vi "Puzzle 24-2.vi"() -> ()   [LabVIEW 2022 SP3]
uses:
  <vilib>/gmath/zero.llb/nD Nonlinear System Solver (Formula).vi
  c09a35fd-dfb7-4751-8a6c-d1f927b46256.vi
  c23b235e-6b21-46d7-9deb-4925a2cb368b.vi
  <vilib>/gmath/NI_Gmath.lvlib
panel:
  in  "delimited string":string="65408297713475, 57213841527206, 185313960119735 @ 316, 321, 204\n185109670669244, 12706941956960, 43641783548659 @ 163, 423, 416\n57063184441840, 2848723329813, 179657077519134 @ 281, 332, 221\n93328649189759, 26248115804612, 49995133784360 @ 290, 377, 390"
  out "sum":dbl
  out "subarray":dbl[][](array[numeric])
  out "f(Zeroes)":dbl[][](array[numeric]) format="%0.2e"
  out "Zeroes 2":dbl[][](array[numeric])
  out "error":i32
  in  "index":i32
  out "Zeroes":dbl[][](array[numeric])
  out "Array":string[](array[string])
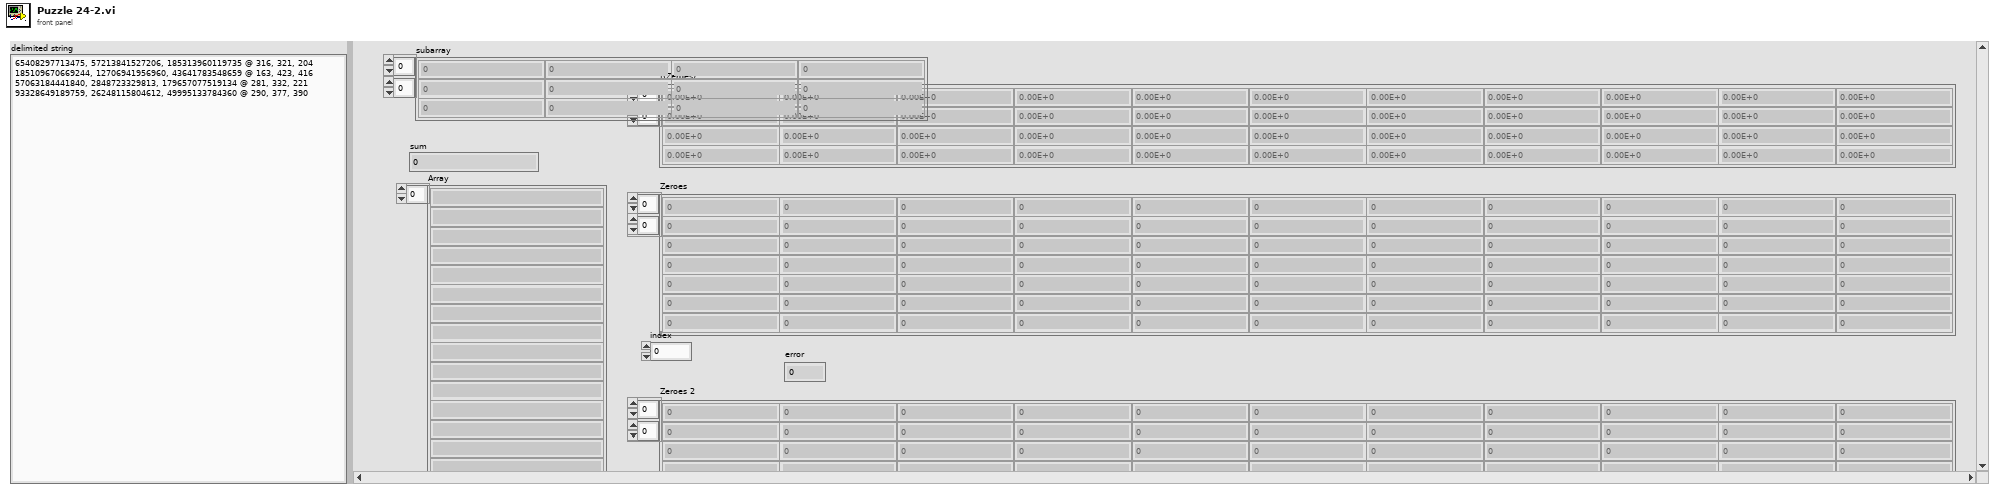
[diagram p1: front panel]
types:
  T1 = cluster{"cluster":cluster{"x":u64, "y":u64, "z":u64}, "cluster":cluster{"x":i64, "y":i64, "z":i64}}
  T2 = cluster{"cluster":cluster{"x":u64, "y":u64, "z":u64}, "cluster":cluster{"x":i64, "y":i64, "z":i64}}[]
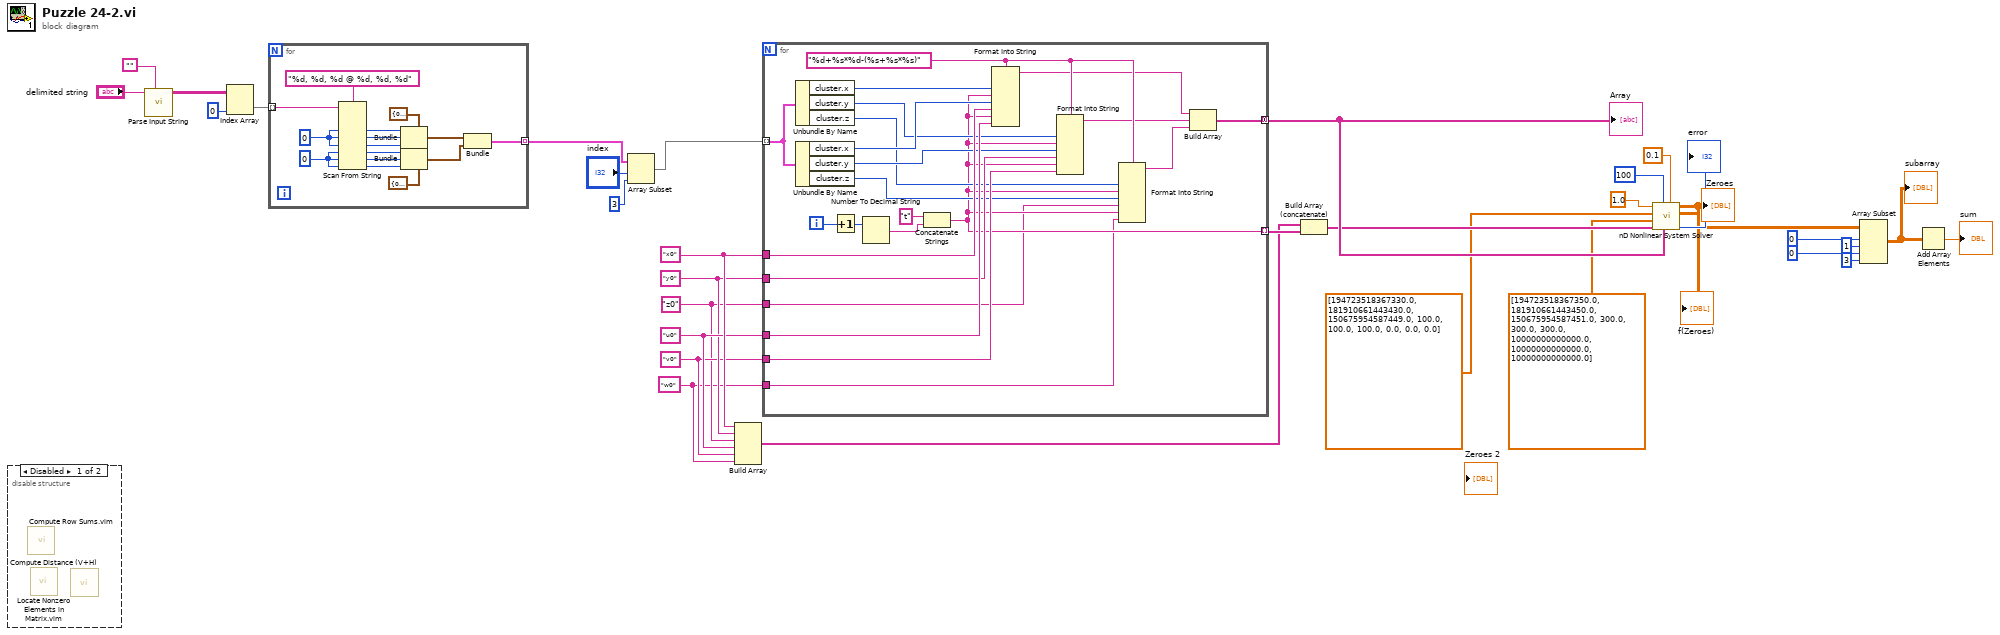
[diagram p0: block diagram]
diagram:
  w22 = "w0" ("string")
  w24 = "v0" ("string")
  w27 = "u0" ("string")
  w23 = "z0" ("string")
  w25 = "y0" ("string")
  w28 = "x0" ("string")
  n1 = disable-structure shown="Disabled" {
    frame Disabled {
      n2 = call "Compute Row Sums.vim"() -> ()  [unwired: 11 in, 1 out]
      n3 = call "Locate Nonzero Elements in Matrix.vim"() -> ()  [unwired: 11 in, 1 out]
      n4 = call "Compute Distance (V+H).vi"() -> ()  [unwired: 11 in, 1 out]
    }
    frame Enabled {
    }
  }
  n5 = call "Parse Input String.vi"("delimiter (Tab)"="", "delimited string"="delimited string") -> ("parsed string"=w32:string[][])  [unwired: 9 in]
  n6 = Index Array(array=w32, index (col)=0 ("disabled index (col)")) -> (element=w30:string[])  [unwired: 1 in]
  n7 = for {
    tunnel: w30 -> [w41] mode=indexing
    tunnel: [w34] -> w15 mode=indexing
    w40 = i64 0 ("default value 1")
    w47 = u64 0 ("default value 1")
    n8 = Scan From String(format string="%d, %d, %d @ %d, %d, %d", input string=w41, default 1=w47, default 2=w47, default 3=w47, default 4=w40, default 5=w40, default 6=w40) -> (output 1=w46:u64, output 2=w45:u64, output 3=w44:u64, output 4=w39:i64, output 5=w38:i64, output 6=w37:i64)  [unwired: 2 in, 3 out]
    n9 = Bundle(cluster=cluster{"x":u64, "y":u64, "z":u64} {"x"=0, "y"=0, "z"=0}, "x"=w46, "y"=w45, "z"=w44) -> (w36:cluster{"x":u64, "y":u64, "z":u64})
    n10 = Bundle(cluster=cluster{"x":i64, "y":i64, "z":i64} {"x"=0, "y"=0, "z"=0}, "x"=w39, "y"=w38, "z"=w37) -> (w35:cluster{"x":i64, "y":i64, "z":i64})
    n11 = Bundle("cluster"=w36, "cluster"=w35) -> (w34:T1)  [unwired: 1 in]
  }
  n12 = Array Subset(array=w15, index="index", length=3) -> (w14:T2)
  n13 = Build Array(w28, w25, w23, w27, w24, w22) -> (w19:string[])
  n14 = for {
    tunnel: w14 -> [w71] mode=indexing
    tunnel: w28 -> [w64]
    tunnel: w27 -> [w63]
    tunnel: [w55] -> w26 mode=indexing
    tunnel: [w49] -> w21 mode=concatenating
    tunnel: w25 -> [w60]
    tunnel: w24 -> [w59]
    tunnel: w23 -> [w54]
    tunnel: w22 -> [w53]
    i -> [w70]
    w58 = "%d+%s*%d-(%s+%s*%s)" ("format string")
    n15 = Unbundle By Name(w71) -> ("cluster.x"=w66:u64, "cluster.y"=w62:u64, "cluster.z"=w57:u64)
    n16 = Unbundle By Name(w71) -> ("cluster.x"=w65:i64, "cluster.y"=w61:i64, "cluster.z"=w56:i64)
    n17 = Increment(x=w70) -> (x+1=w69:i32)
    n18 = Number To Decimal String(number=w69) -> (decimal integer string=w67:string)  [unwired: 1 in]
    n19 = Concatenate Strings("t" ("string"), w67) -> (w55:string)
    n20 = Format Into String(format string=w58, w66, w55, w65, w64, w55, w63) -> (resulting string=w52:string)  [unwired: 2 in, 1 out]
    n21 = Format Into String(format string=w58, w62, w55, w61, w60, w55, w59) -> (resulting string=w51:string)  [unwired: 2 in, 1 out]
    n22 = Format Into String(format string=w58, w57, w55, w56, w54, w55, w53) -> (resulting string=w50:string)  [unwired: 2 in, 1 out]
    n23 = Build Array(w52, w51, w50) -> (w49:string[])
  }
  "Array" <- w21
  n24 = Build Array (concatenate)(w19, w26) -> (w18:string[])
  n25 = call-poly <vilib>:"nD Nonlinear System Solver.vi"("accuracy"=0.1, "F(X)"=w21, "number of trials"=u32 100, "X"=w18, "End"=dbl[] [194723518367350.0, 181910661443450.0, 150675954587451.0, 300.0, 300.0, 300.0, 10000000000000.0, 10000000000000.0, 10000000000000.0] ("initialized array"), "Start"=dbl[] [194723518367330.0, 181910661443430.0, 150675954587449.0, 100.0, 100.0, 100.0, 0.0, 0.0, 0.0] ("initialized array"), "h"=1.0) -> ("error"=→"error":i32, "f(Zeroes)"=→"f(Zeroes)":dbl[][], "Zeroes"=w7:dbl[][])  [unwired: 1 in, 1 out]
  "Zeroes" <- w7
  n26 = Array Subset(array=w7, index (row)=0 ("index"), length (row)=1 ("length"), index (col)=0 ("index"), length (col)=3 ("length")) -> (w2:dbl[][])
  "subarray" <- w2
  n27 = Add Array Elements(numeric array=w2) -> (sum=→"sum":dbl)
